vi "_password_db.vi"(6 "Enum":T3, 8 "Error in":errorcluster caption="Error in (no error)", 11 "Userinfo":T1={"UserName"="", "Password"="", "Role"=enum."Admin"}) -> (0 "Error out":errorcluster, 1 "appended array":T1[](array[typedef]), 2 "Boolean":bool, 3 "Userinfo (dup)":T1={"UserName"="", "Password"="", "Role"=enum."Admin"})   [LabVIEW 2017, in "Login-UI.lvlib"]
uses:
  Login-UI.lvlib
  _Typedef/User-Info.ctl
  _Typedef/User-Role.ctl
  _password_db_oper.ctl
  de08a50a-4147-4a78-afe1-ead21049d83f.vi
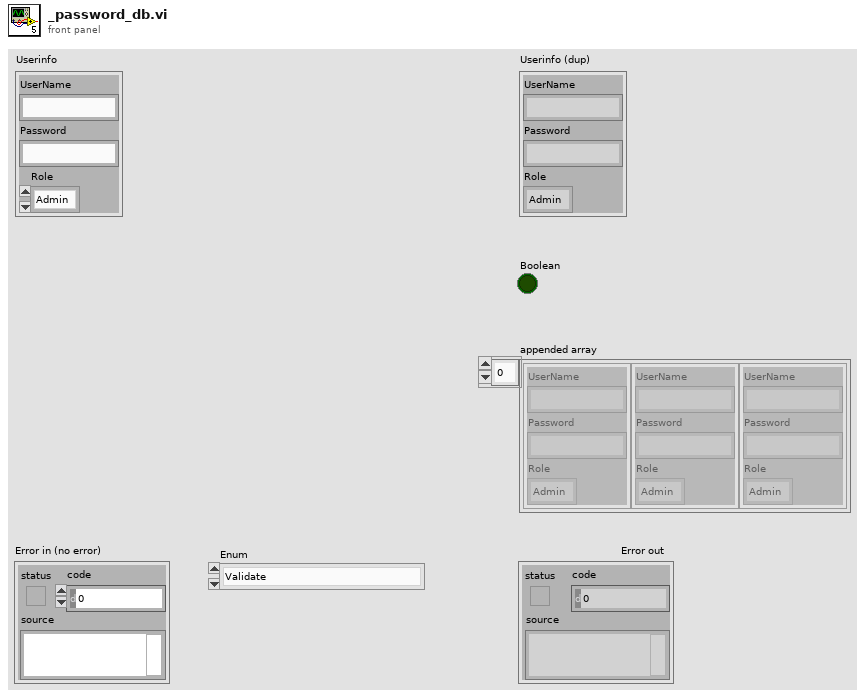
[diagram p1: front panel]
types:
  T1 = typedef "Login-UI.lvlib/User-Info.ctl" = cluster{"UserName":string, "Password":string, "Role":T2}
  T2 = typedef "Login-UI.lvlib/User-Role.ctl" = enum16{"INVALID", "Operator", "Engineer", "Admin", "Anonymous"}
  T3 = typedef "Login-UI.lvlib/_password_db_oper.ctl" = enum16{"Validate", "Register", "Unregister", "View"}
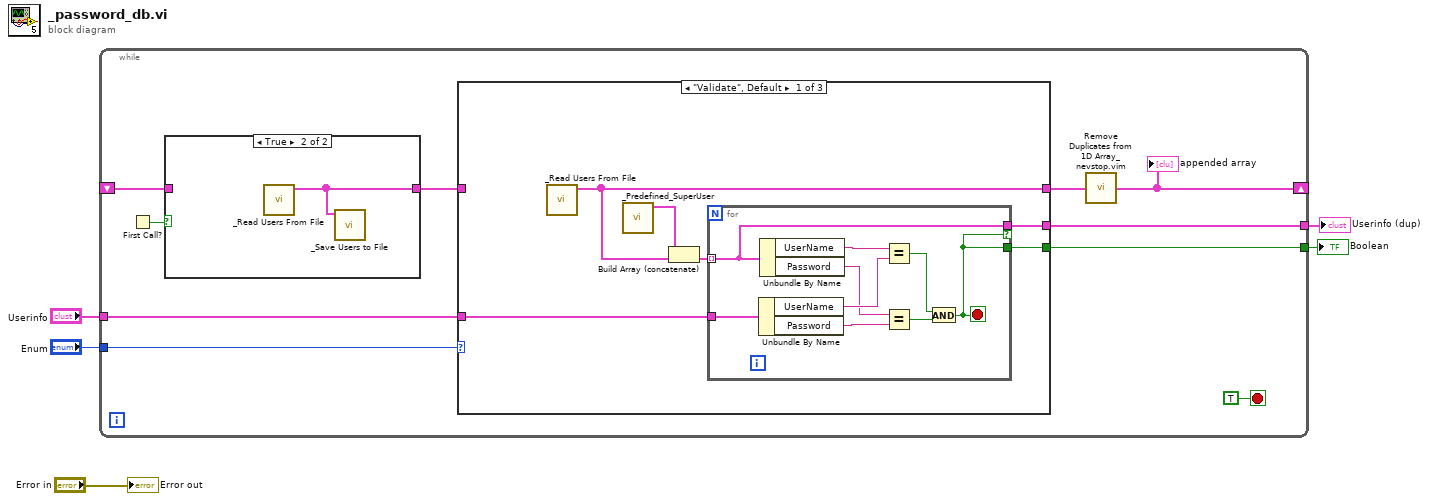
[diagram p0: block diagram]
diagram:
  n1 = while {
    shift-right: [w6] -> _
    shift-left: _ -> [w12]
    tunnel: "Enum" -> [w10]
    tunnel: "Userinfo" -> [w9]
    tunnel: [w8] -> w2
    tunnel: [w7] -> w1
    stop <- TRUE stop-if-true
    n2 = First Call?() -> (First Call?: T/F=w13:bool)
    n3 = case shown="True" w13 {
      tunnel: [w16 w17] -> w14
      tunnel: w12 -> [w16 _]
      frame False {
      }
      frame True {
        n4 = call "_Read Users From File.vi"() -> ("Array"=w17:T1[])  [unwired: 10 in, 1 out]
        n5 = call "_Save Users to File.vi"("Array"=w17) -> ()  [unwired: 10 in, 1 out]
      }
    }
    n6 = case shown="\"Validate\", Default" w10 {
      tunnel: [w18 w33 w34] -> w11
      tunnel: w14 -> [_ w33 w34]
      tunnel: w9 -> [w23 _ _]
      tunnel: [w22 _ _] -> w8
      tunnel: [w21 _ _] -> w7
      frame "Validate", Default {
        n7 = call "_Read Users From File.vi"() -> ("Array"=w18:T1[])  [unwired: 10 in, 1 out]
        n8 = call "_Predefined_SuperUser.vi"() -> ("SuperUsers"=w19:T1[])  [unwired: 11 in]
        n9 = Build Array (concatenate)(w19, w18) -> (w20:T1[])
        n10 = for {
          tunnel: w20 -> [w25] mode=indexing
          tunnel: w23 -> [w32]
          tunnel: [w24] -> w22
          tunnel: [w25] -> w21 if=w24
          stop <- w24 stop-if-true
          n11 = Unbundle By Name(w32) -> ("UserName"=w30:string, "Password"=w29:string)
          n12 = Unbundle By Name(w25) -> ("UserName"=w31:string, "Password"=w28:string)
          n13 = Equal?(x=w31, y=w30) -> (x = y?=w26:bool)
          n14 = Equal?(x=w28, y=w29) -> (x = y?=w27:bool)
          n15 = And(x=w26, y=w27) -> (x .and. y?=w24:bool)
        }
      }
      frame "View" {
      }
      frame "Register" {
      }
    }
    n16 = call "Remove Duplicates from 1D Array_nevstop.vim"("Input Array"=w11) -> ("Output Array"=w6:T1[])  [unwired: 1 out]
    "appended array" <- w6
  }
  "Boolean" <- w2
  "Userinfo (dup)" <- w1
  "Error out" <- "Error in"
